vi "RWDI.vi"(4 "Freq":dbl[](array[numeric]), 5 "Phase In":dbl[](array[numeric]), 6 "Magnitude In":dbl[](array[numeric]), 7 "Tranfer_Function_File":path) -> (1 "Phase Out":dbl[](array[numeric]), 2 "Magnitude Out":dbl[](array[numeric]))   [LabVIEW 2011]
uses:
  <vilib>/Utility/file.llb/Read From Spreadsheet File (DBL).vi
  <vilib>/Analysis/NI_AALPro.lvlib
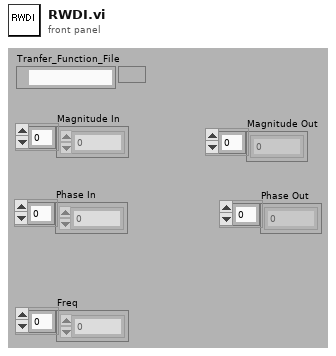
[diagram p1: front panel]
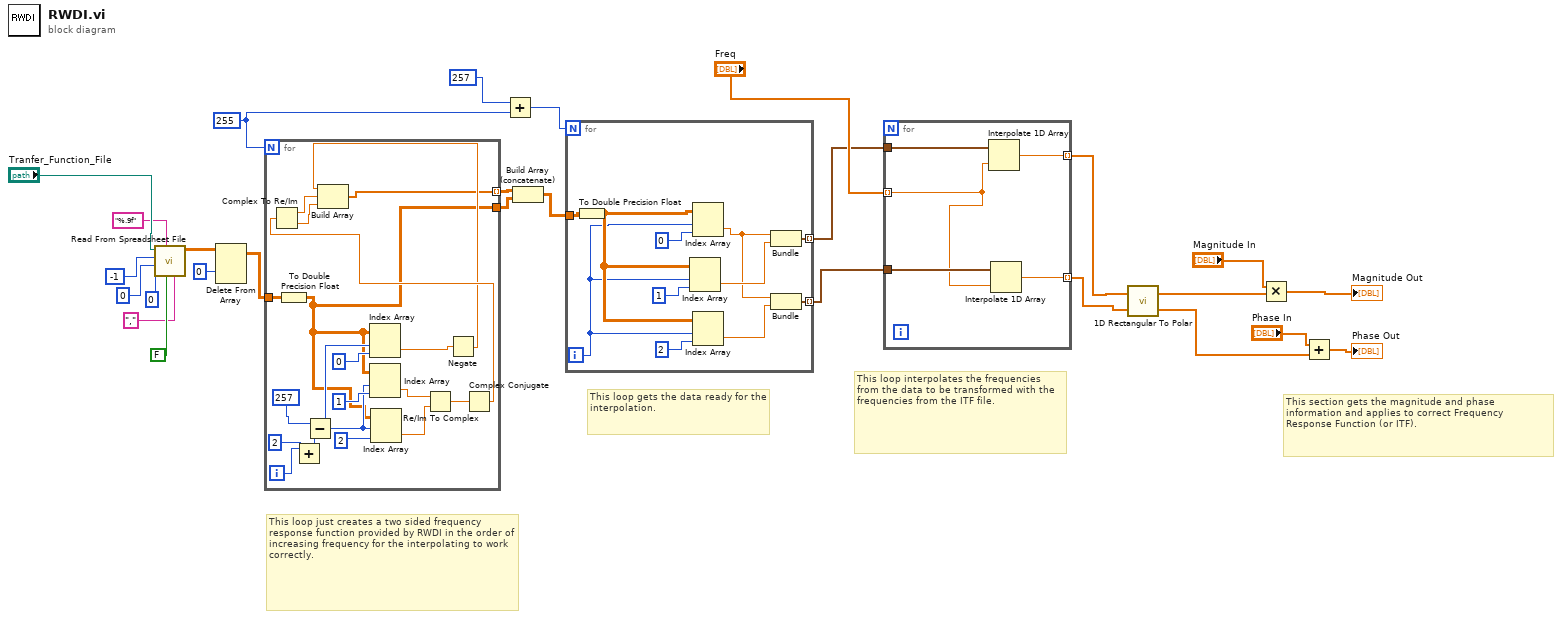
[diagram p0: block diagram]
diagram:
  w18 = 255
  # "This section gets the magnitude and phase information and applies to correct Frequency Response Function (or ITF)."
  # "This loop interpolates the frequencies from the data to be transformed with the frequencies from the ITF file."
  # "This loop gets the data ready for the interpolation."
  # "This loop just creates a two sided frequency response function provided by RWDI in the order of increasing frequency for the interpolating to work correctly."
  n1 = call-poly <vilib>:"Read From Spreadsheet File.vi"("delimiter (\\t)"="," ("delimiter (Tab)"), "transpose (no:F)"=FALSE, "format (%.3f)"="%.9f", "max characters/row  (no limit:0)"=0, "start of read offset (chars.:0)"=0, "number of rows (all:-1)"=-1, "file path (dialog if empty)"="Tranfer_Function_File") -> ("all rows"=w7:dbl[][])  [unwired: 4 out]
  n2 = Delete From Array(array=w7, index (row)=0) -> (array with subset deleted=w16:dbl[][])  [unwired: 2 in, 1 out]
  n3 = for {
    N: w18 -> [_]
    tunnel: w16 -> [w46]
    tunnel: [w29] -> w20 mode=indexing
    tunnel: [w28] -> w21
    i -> [w32]
    n4 = To Double Precision Float(number=w46) -> (double precision float=w28:dbl[][])
    n5 = Add(x=w32, y=2 ("disabled index (col)")) -> (x+y=w40:i32)
    n6 = Subtract(x=257, y=w40) -> (x-y=w39:i32)
    n7 = Index Array(array=w28, index (row)=w39, index (col)=0 ("disabled index (col)")) -> (element=w31:dbl)
    n8 = Index Array(array=w28, index (row)=w39, index (col)=1 ("disabled index (col)")) -> (element=w38:dbl)
    n9 = Index Array(array=w28, index (row)=w39, index (col)=2 ("disabled index (col)")) -> (element=w37:dbl)
    n10 = Re/Im To Complex(1:w37, 2:w38) -> (0:w36:cdb)
    n11 = Negate(x=w31) -> (-x=w30:dbl)
    n12 = Complex Conjugate(1:w36) -> (0:w35:cdb)
    n13 = Complex To Re/Im(x + iy=w35) -> (x=w34:dbl, y=w33:dbl)
    n14 = Build Array(w30, w34, w33) -> (w29:dbl[])
  }
  n15 = Add(x=257, y=w18) -> (x+y=w19:i32)
  n16 = Build Array (concatenate)(w20, w21) -> (w22:dbl[][])
  n17 = for {
    N: w19 -> [_]
    tunnel: w22 -> [w57]
    tunnel: [w49] -> w10 mode=indexing
    tunnel: [w47] -> w9 mode=indexing
    i -> [w48]
    n18 = To Double Precision Float(number=w57) -> (double precision float=w53:dbl[][])
    n19 = Index Array(array=w53, index (row)=w48, index (col)=1 ("disabled index (col)")) -> (element=w52:dbl)
    n20 = Index Array(array=w53, index (row)=w48, index (col)=0 ("disabled index (col)")) -> (element=w51:dbl)
    n21 = Index Array(array=w53, index (row)=w48, index (col)=2 ("disabled index (col)")) -> (element=w50:dbl)
    n22 = Bundle(w51, w52) -> (w49:cluster{dbl, dbl})  [unwired: 1 out]
    n23 = Bundle(w51, w50) -> (w47:cluster{dbl, dbl})  [unwired: 1 out]
  }
  n24 = for {
    tunnel: w9 -> [w62]
    tunnel: w10 -> [w61]
    tunnel: "Freq" -> [w58] mode=indexing
    tunnel: [w60] -> w26 mode=indexing
    tunnel: [w59] -> w27 mode=indexing
    n25 = Interpolate 1D Array(1:w58, 2:w61) -> (0:w60:dbl)
    n26 = Interpolate 1D Array(1:w58, 2:w62) -> (0:w59:dbl)
  }
  n27 = call <vilib>:"1D Rectangular To Polar.vi"("X"=w26, "Y"=w27) -> ("Magnitude"=w11:dbl[], "Phase"=w23:dbl[])  [unwired: 1 out]
  n28 = Multiply(x="Magnitude In", y=w11) -> (x*y=→"Magnitude Out":dbl[])
  n29 = Add(x="Phase In", y=w23) -> (x+y=→"Phase Out":dbl[])
